vi "19052 Initialize with retry.vi"(6 "Retry settings":cluster{"TBR (s)":u32, "MRA":i32}={"TBR (s)"=1, "MRA"=10} {"MRA" min=1 max=100 step=1; "TBR (s)" max=100 step=1}, 7 "Serial Configuration":T1={"Baud Rate"=9600, "Flow Control"=0, "Parity"=0, "Data Bits"=8} {"Baud Rate" items=["300"=300, "600"=600, "1200"=1200, "2400"=2400, "4800"=4800, "9600"=9600, "19200"=19200]; "Flow Control" items=["NONE", "SOFTWARE"]; "Parity" items=["NONE", "ODD", "EVEN"]; "Data Bits" items=["7"=7, "8"=8]}, 8 "error in (no error)":errorcluster, 9 "Reset (True)":bool=TRUE, 10 "ID Query (True)":bool=TRUE, 11 "VISA resource name":refnum<visa-resource-name>) -> (0 "error out":errorcluster, 2 "Message":string, 3 "VISA resource name out":refnum<visa-resource-name>)   [LabVIEW 2025]
doc: "This VI is a wrapper for the instrument initialization process. It attempts to establish a VISA session with the specified resource name, including configurable retry logic. If initialization fails, the VI retries according to the specified settings and generates detailed error messages with timestamps for each attempt.\n\n<b>Inputs:</b>\n<b>Retry Settings (Cluster):</b>\n<b>TBR (U32):</b> Time Between Retries, in seconds.\n<b>MRA (U32):</b> Maximum number of Retry Attempts.\n<b>Serial Configuration (Cluster):</b> Serial port settings when using RS-232.\n<b>VISA Resource Name (String):</b> Identifies the instrument resource to connect to.\n<b>ID Query (Boolean):</b> If TRUE, performs an identification query during initialization.\n<b>Reset (Boolean):</b> If TRUE, sends a device reset command during initialization.\n<b>Error In (Cluster):</b> Propagates errors from previous VIs.\n\n<b>Outputs:</b>\n<b>VISA Resource Name Out (String):</b> Returns the VISA resource actually used for the connection.\n<b>Message (String):</b> Log text with results of each attempt (try number, timestamp, and error description if any).\n<b>Error Out (Cluster):</b> Reports error status, code, and source description."
uses:
  <vilib>/Utility/error.llb/DialogType.ctl
  <instrlib>/Chroma 19052/Chroma 19052.lvlib
panel:
  # "Retry settings:\nTBR = Time Between Retries (sec)\nMRA = Maximum Retry Attempts"
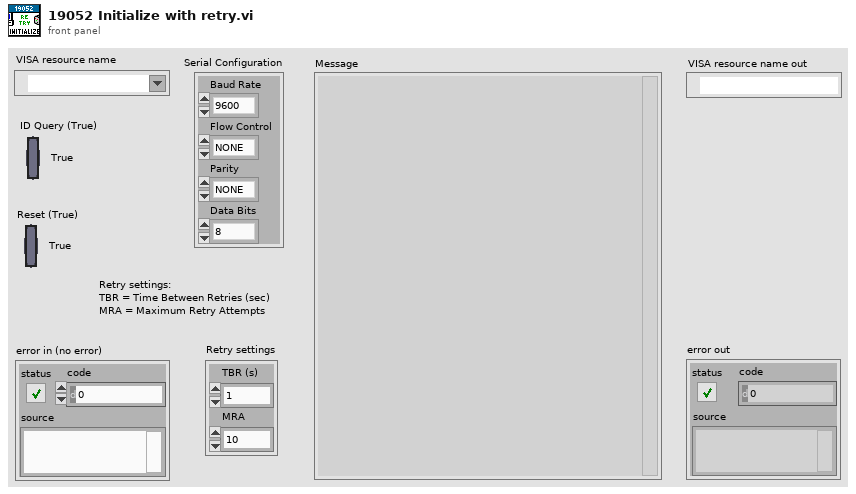
[diagram p1: front panel]
types:
  T1 = cluster{"Baud Rate":u32, "Flow Control":u16, "Parity":u16, "Data Bits":u16}
  T2 = typedef "DialogType.ctl" = u16
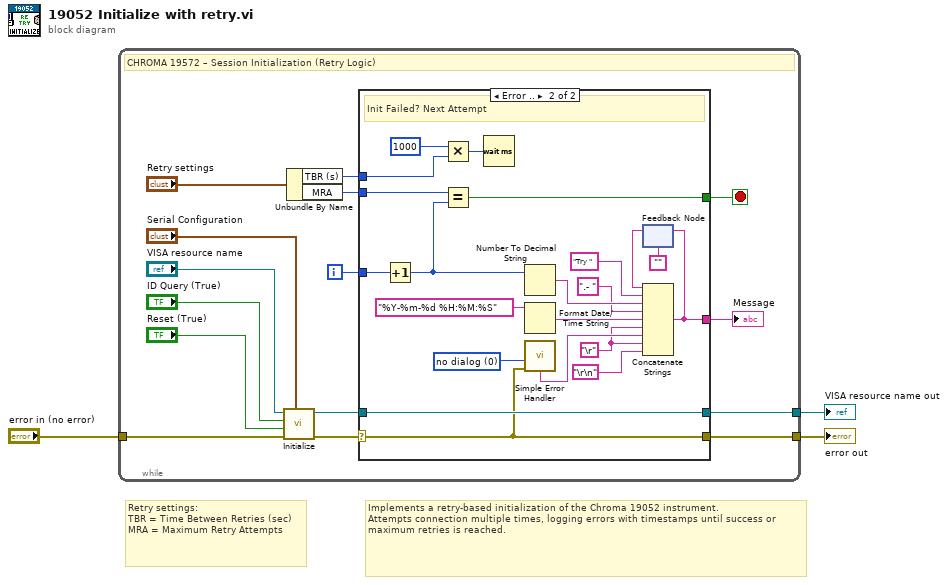
[diagram p0: block diagram]
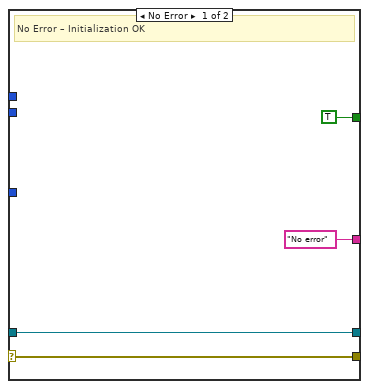
[diagram p2: hidden frame]
diagram:
  # "Implements a retry-based initialization of the Chroma 19052 instrument.\nAttempts connection multiple times, logging errors with timestamps until success or maximum retries is reached."
  # "Retry settings:\nTBR = Time Between Retries (sec)\nMRA = Maximum Retry Attempts"
  n1 = while {
    tunnel: [w14] -> w2
    tunnel: "error in (no error)" -> [w13]
    tunnel: [w12] -> w3
    i -> [w17]
    stop <- w16 stop-if-true
    # "CHROMA 19572 – Session Initialization (Retry Logic)"
    n2 = call <instrlib>:"Initialize.vi"("Serial Configuration"="Serial Configuration", "error in (no error)"=w13, "Reset (True)"="Reset (True)", "ID Query (True)"="ID Query (True)", "VISA resource name"="VISA resource name") -> ("error out"=w18:errorcluster, "VISA resource name out"=w15:refnum<visa-resource-name>)  [unwired: 5 in]
    n3 = Unbundle By Name("Retry settings") -> ("TBR (s)"=w9:u32, "MRA"=w10:i32)
    n4 = case shown="Error .." w18 {
      selector: w18 -> [w22 w26]
      tunnel: [w22 w26] -> w12
      tunnel: w17 -> [_ w39]
      tunnel: [TRUE w40] -> w16
      tunnel: w15 -> [w20 w42]
      tunnel: [w20 w42] -> w14
      tunnel: ["No error" w25] -> w11
      tunnel: w10 -> [_ w34]
      tunnel: w9 -> [_ w32]
      frame No Error {
        # "No Error – Initialization OK"
      }
      frame Error {
        w29 = "\r" ("Carriage Return Constant")
        w41 = T2 0 items=["no dialog", "OK message", "continue or stop message", "OK message + warnings", "continue/stop + warnings"] ("type of dialog (OK msg:1)")
        # "Init Failed? Next Attempt"
        n5 = Increment(x=w39) -> (x+1=w35:i32)
        n6 = Multiply(x=u32 1000 ("y"), y=w32) -> (x*y=w33:u32)
        n7 = Equal?(x=w34, y=w35) -> (x = y?=w40:bool)
        n8 = Wait (ms)(milliseconds to wait=w33) -> ()  [unwired: 1 out]
        n9 = Number To Decimal String(number=w35) -> (decimal integer string=w38:string)  [unwired: 1 in]
        n10 = Format Date/Time String(time format string (%c)="%Y-%m-%d %H:%M:%S") -> (date/time string=w27:string)  [unwired: 2 in]
        n11 = call <vilib>:"Simple Error Handler.vi"("type of dialog (OK msg:1)"=w41, "error in (no error)"=w26) -> ("message"=w43:string)  [unwired: 3 in, 4 out]
        n12 = feedback #1("" ("Empty String Constant")) -> (w24:string)
        n13 = Concatenate Strings(w24, "Try " ("string"), w38, ".- " ("string"), w27, w29, w43, w29, "\r\n" ("End of Line Constant")) -> (w25:string)
        n14 = feedback-in #1(w25) -> ()
      }
    }
    "Message" <- w11
  }
  "VISA resource name out" <- w2
  "error out" <- w3
